vi "Scripts.vi"() -> ()   [LabVIEW 2013]
uses:
  <vilib>/Platform/TimedLoop/XDataNode/wakeup.ctl
  <vilib>/Platform/TimedLoop/XDataNode/XDNodeRunTimeDep.lvlib
  <vilib>/Platform/TimedLoop/XDataNode/nitl_modes.ctl
  <vilib>/Platform/TimedLoop/XDataNode/timing_clust.ctl
  <vilib>/Platform/TimedLoop/XDataNode/XDataNode.xnode
panel:
  in  "Stop All":bool=TRUE
  in  "Green Laser ON/Interlacing":bool
  in  "Green laser mode":enum32{"Laser ON", "Laser OFF", "Interlace"}(radio)
  in  "Green FB On/Off":bool
  in  "Stop Saving":bool
  in  "Fl. Triggered...":bool
  out "Tether":bool
  in  "Save ave N":dbl=500.0 caption="Averaging Factor"
  out "Raster Scanning...":bool
  out "Saving...":bool
  out "Stage Moving":bool
  in  "Take Detection Laser\nImage":bool
  in  "Step Size (nm)":dbl=0.34
  in  "N Steps":dbl=20.0
  in  "Take Stepping Data":bool
  in  "Save ave factor":dbl=1.0
  in  "Got DNA bead":bool
  in  "Got ADig bead":bool
  in  "Y change (mm)":dbl
  in  "Dip for Protein":bool
  in  "Save Data After?":bool
  in  "Green ON After?":bool
  in  "Dip Trap Delta 2 (MHz)":dbl=15.0
  in  "Move Trap After?":bool
  in  "Duration (s)":dbl=1.0
  in  "Move Trap Before?":bool
  in  "Dip Trap Delta 1 (MHz)":dbl=15.0
  in  "Dump Beads":bool
  in  "Cal/Data Acq. Spot":bool
  in  "Offset 2 Start (MHz)":dbl=16.0
  in  "Offset 2 Set":dbl=2.0
  in  "Cal read wait (s)":u32=5
  in  "W/ Offset 2":bool
  in  "Offset 1 Start (MHz)":dbl=13.0
  in  "Offset 1 Set":dbl=1.0
  in  "W/ Offset 1":bool=TRUE
  in  "Cal @ (MHz)":dbl=20.0
  in  "Cap 1 T ON":bool=TRUE
  in  "Cap 1 Flow ON":bool=TRUE
  in  "Move Cap. 1 (DNA Top)":bool
  in  "Cap 1 Samp Flow ON":bool=TRUE
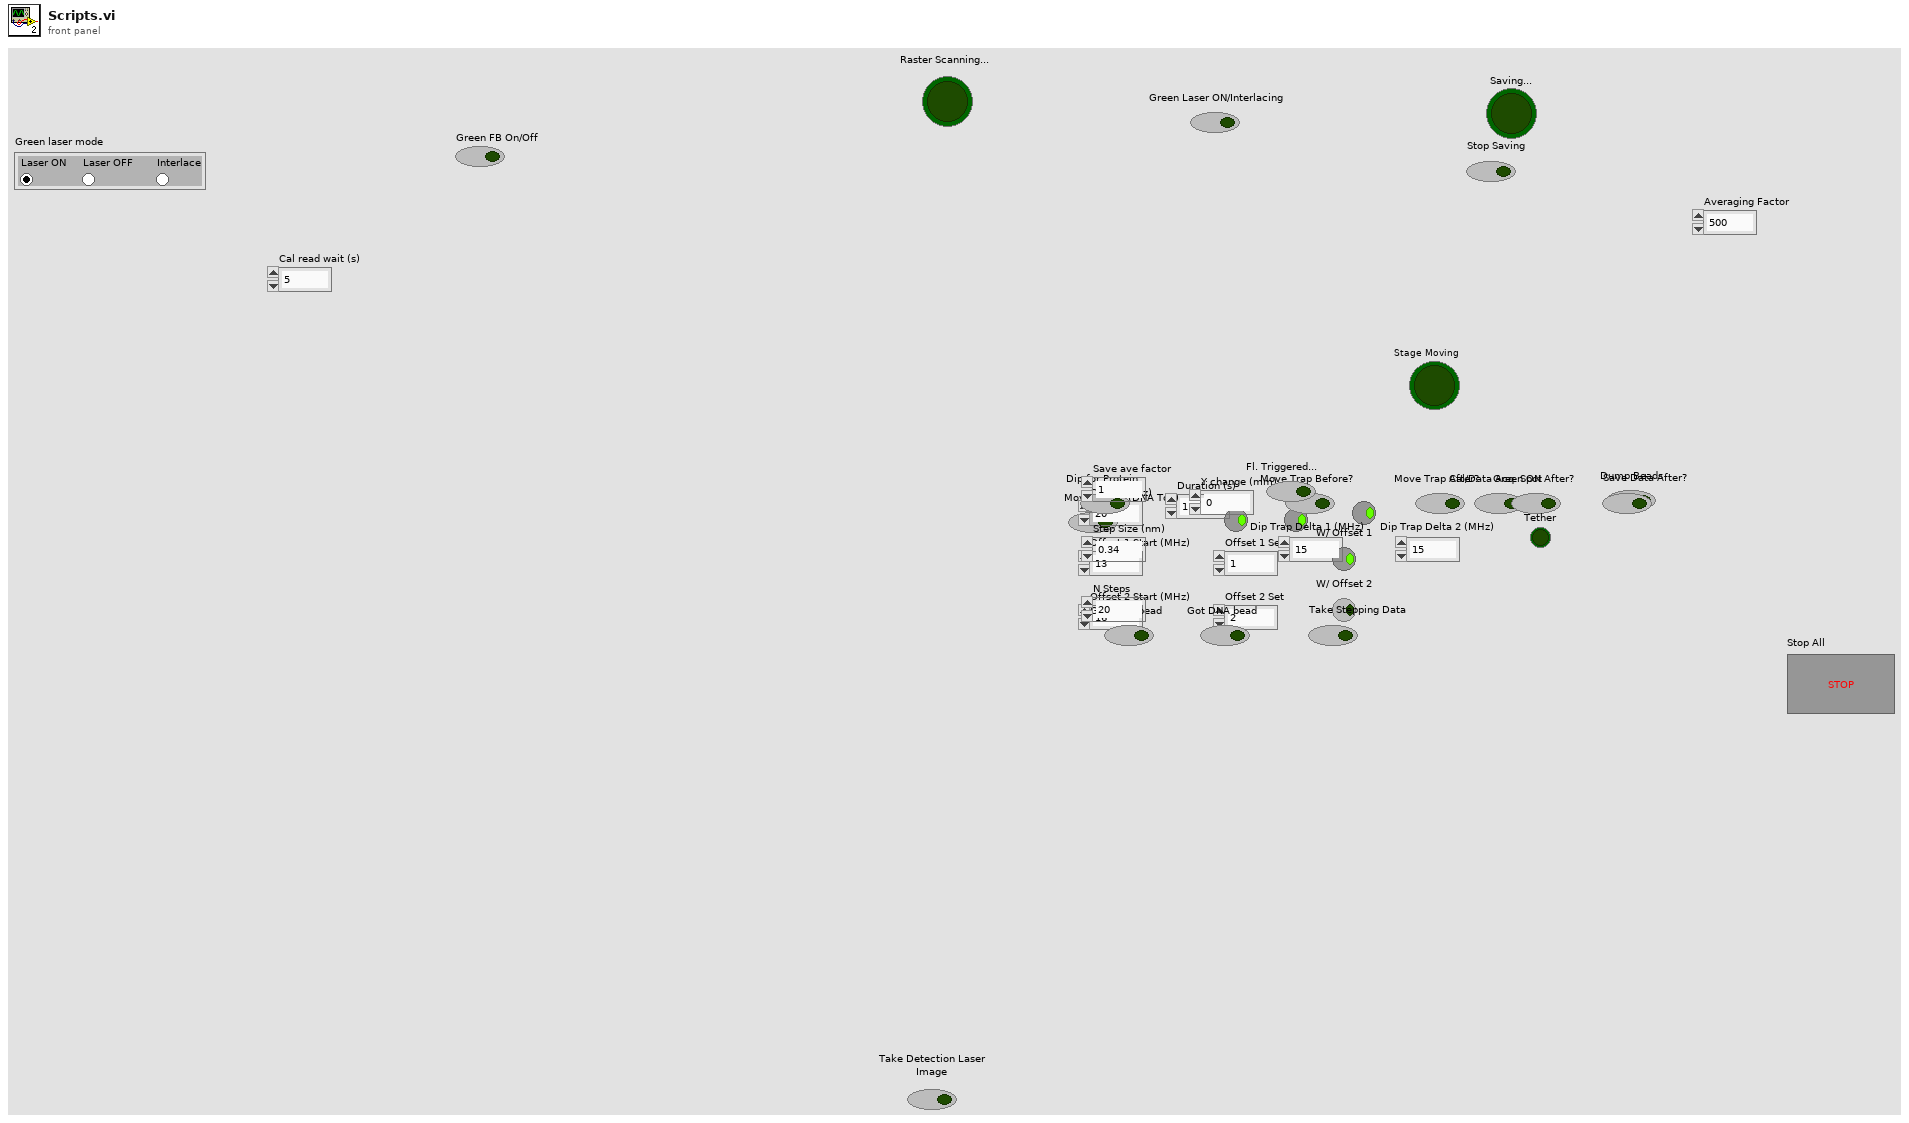
[diagram p1: front panel]
types:
  T1 = typedef "XDNodeRunTimeDep.lvlib/timing_clust.ctl" = cluster{"Expected End [f-1]":u64, "Actual End [f-1]":u64, "Finished Late? [f-1]":bool, "Expected End [i-1]":u64, "Actual End [i-1]":u64, "Finished Late? [i-1]":bool, "Expected Start [i]":u64, "Actual Start [i]":u64, "Expected Start [f]":u64, "Actual Start [f]":u64, "Source Name":string, "Structure Name":string, "Period":i64, "Deadline":i64, "Offset":i64, "Start":i64, "Priority":i32, "Timeout":i32, "Mode":T2, "Wakeup Reason":T3, "Error":errorcluster, "Source Type":string, "Secondary Source Type":string, "Global End Time":u64, "Global Start Time":u64, "Frame Duration":u64, "Iteration Duration":u64, "Assigned CPU":i32, "I/O Scan Engine Mode":u32}
  T2 = typedef "XDNodeRunTimeDep.lvlib/nitl_modes.ctl" = enum32{"No Change", "Process missed periods, maintain original phase", "Discard missed periods, maintain original phase", "Process missed periods, ignore original phase", "Discard missed periods, ignore original phase"}
  T3 = typedef "XDNodeRunTimeDep.lvlib/wakeup.ctl" = enum32{"Normal", "Aborted", "Asynchronous wakeup", "Timing source error", "Timed loop error", "Timeout"}
  T4 = enum16{"CONNECT", "INITIALIZE VALVES", "DISCONNECT", "MOVE VALVE"}
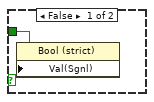
[diagram p4: hidden frame]
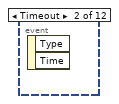
[diagram p5: hidden frame]
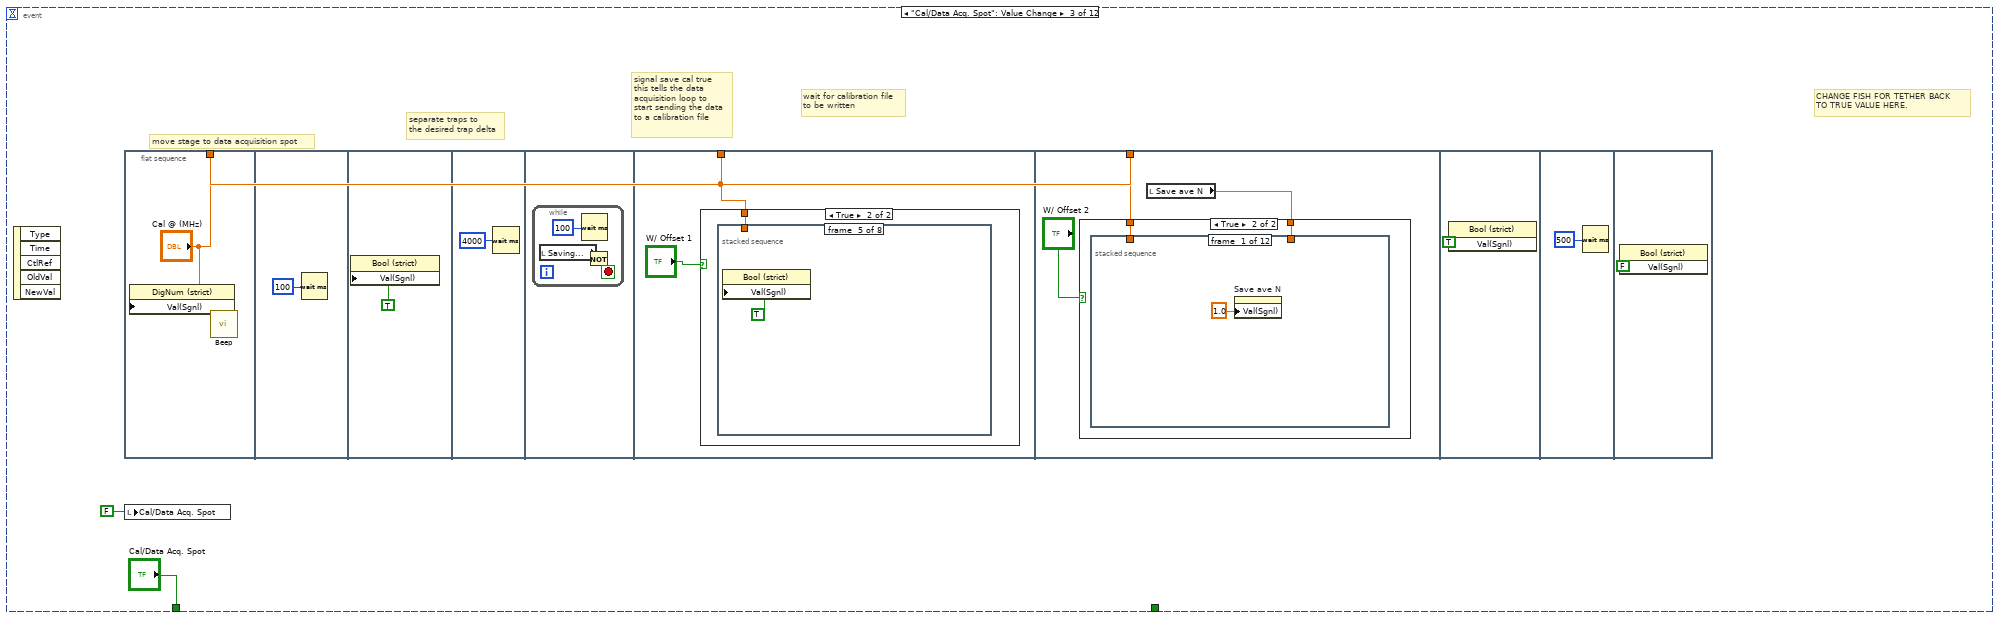
[diagram p6: hidden frame]
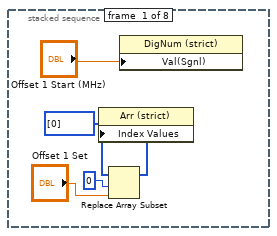
[diagram p8: hidden frame]
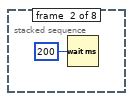
[diagram p9: hidden frame]
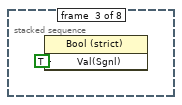
[diagram p10: hidden frame]
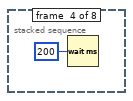
[diagram p11: hidden frame]
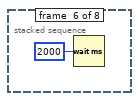
[diagram p12: hidden frame]
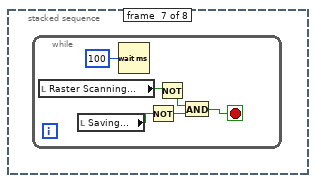
[diagram p13: hidden frame]
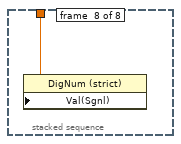
[diagram p14: hidden frame]
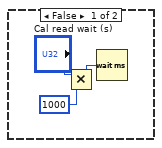
[diagram p15: hidden frame]
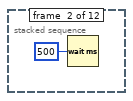
[diagram p16: hidden frame]
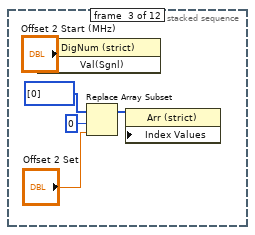
[diagram p17: hidden frame]
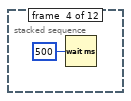
[diagram p18: hidden frame]
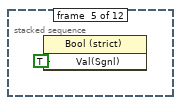
[diagram p19: hidden frame]
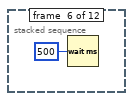
[diagram p20: hidden frame]
diagram:
  n1 = node-c288() -> (w2:T1)  [unwired: 4 in]
  n2 = timed-loop "Run Scripts, including: stage motion" {
    timing: w2 -> [_]
    timing-out: [_] -> w1
    stop <- w4 stop-if-true
    n3 = node-c288() -> ()  [unwired: 1 in, 1 out]
    n4 = event shown="[0] \"Move Cap. 1 (DNA Top)\": Value Change" {
      selector: _ -> [_ _ _ _ _ _ _ _ _ _ _ _]
      dyn-events: _ -> [_ _ _ _ _ _ _ _ _ _ _ _]
      timeout: 50 -> [_ _ _ _ _ _ _ _ _ _ _ _]
      tunnel: ["Move Cap. 1 (DNA Top)" _ "Cal/Data Acq. Spot" "Dump Beads" "Dip for Protein" _ "Got ADig bead" "Got DNA bead" "Take Stepping Data" _ "Take Detection Laser\nImage" _] -> _
      tunnel: [_ _ _ _ _ _ _ _ _ _ _ w212] -> w4
      event "Move Cap. 1 (DNA Top)": Value Change {
        n5 = event-data() -> ()  [unwired: 1 in, 5 out]
        n6 = local write "Move Cap. 1 (DNA Top)"(FALSE ("Move Cap. 1 (DNA Right)")) -> ()
        n7 = flat-sequence {
          tunnel: "Cap 1 Samp Flow ON" -> [w10]
          frame #0 {
            n8 = local write "Stage Moving"(FALSE ("Stage Moving")) -> ()
            n9 = case "stop flow" shown="True" w10 {
              frame False {
              }
              frame True {
                n10 = call "hamilton_controller.vi"("Open?"=FALSE, "valve"=enum16{"A", "B", "C", "D", "ALL"}."C", "action"=T4."MOVE VALVE") -> ()  [unwired: 8 in, 1 out]
              }
            }
            n11 = case shown="True" TRUE {
              tunnel: "Cap 1 T ON" -> [w19 w20]
              frame False {
                n12 = property on="Property Node" class="Bool (strict)"("Val(Sgnl)"=w19) -> ()  [unwired: 2 in, 2 out]
              }
              frame True {
                n13 = property on="Property Node" class="Bool (strict)"("Val(Sgnl)"=w20) -> ()  [unwired: 2 in, 2 out]
              }
            }
            n14 = call <vilib>:"Beep.vi"() -> ()  [unwired: 3 in, 9 out]
            n15 = case shown="True" "Cap 1 Flow ON" {
              frame False {
              }
              frame True {
                n16 = property on="Property Node" class="Bool (strict)"("Val(Sgnl)"=TRUE ("Value (Signaling)")) -> ()  [unwired: 2 in, 2 out]
              }
            }
          }
        }
      }
      event Timeout {
        n17 = event-data() -> ()  [unwired: 1 in, 2 out]
      }
      event "Cal/Data Acq. Spot": Value Change {
        # "wait for calibration file\nto be written"
        # "signal save cal true\nthis tells the data \nacquisition loop to\nstart sending the data\nto a calibration file"
        # "separate traps to\nthe desired trap delta"
        # "move stage to data acquisition spot"
        # "CHANGE FISH FOR TETHER BACK\nTO TRUE VALUE HERE."
        n18 = event-data() -> ()  [unwired: 1 in, 5 out]
        n19 = flat-sequence {
          tunnel: ["Cal @ (MHz)"] -> w21
          tunnel: w21 -> [w31]
          tunnel: w21 -> [w52]
          frame #0 {
            n20 = property on="Property Node" class="DigNum (strict)"("Val(Sgnl)"="Cal @ (MHz)") -> ()  [unwired: 2 in, 2 out]
            n21 = call <vilib>:"Beep.vi"() -> ()  [unwired: 3 in, 9 out]
          }
          frame #1 {
            n22 = Wait (ms)(milliseconds to wait=u32 100) -> ()  [unwired: 1 out]
          }
          frame #2 {
            n23 = property on="Property Node" class="Bool (strict)"("Val(Sgnl)"=TRUE ("Value (Signaling)")) -> ()  [unwired: 2 in, 2 out]
          }
          frame #3 {
            n24 = Wait (ms)(milliseconds to wait=u32 4000) -> ()  [unwired: 1 out]
          }
          frame #4 {
            n25 = while {
              stop <- w28 stop-if-true
              n26 = local read "Saving..."() -> (w29:bool)
              n27 = Wait (ms)(milliseconds to wait=u32 100) -> ()  [unwired: 1 out]
              n28 = Not(x=w29) -> (.not. x?=w28:bool)
            }
          }
          frame #5 {
            n29 = case shown="True" "W/ Offset 1" {
              tunnel: w31 -> [_ w33]
              frame False {
              }
              frame True {
                n30 = stacked-sequence {
                  tunnel: w33 -> [_ _ _ _ _ _ _ w50]
                  frame #0 {
                    n31 = Replace Array Subset(array=u32[] [0] ("Index Values"), new element="Offset 1 Set", index=0) -> (w34:u32[])
                    n32 = property on="Property Node" class="Arr (strict)"("Index Values"=w34) -> ()  [unwired: 2 in, 2 out]
                    n33 = property on="Property Node" class="DigNum (strict)"("Val(Sgnl)"="Offset 1 Start (MHz)") -> ()  [unwired: 2 in, 2 out]
                  }
                  frame #1 {
                    n34 = Wait (ms)(milliseconds to wait=u32 200) -> ()  [unwired: 1 out]
                  }
                  frame #2 {
                    n35 = property on="Property Node" class="Bool (strict)"("Val(Sgnl)"=TRUE ("Value (Signaling)")) -> ()  [unwired: 2 in, 2 out]
                  }
                  frame #3 {
                    n36 = Wait (ms)(milliseconds to wait=u32 200) -> ()  [unwired: 1 out]
                  }
                  frame #4 {
                    n37 = property on="Property Node" class="Bool (strict)"("Val(Sgnl)"=TRUE ("Value (Signaling)")) -> ()  [unwired: 2 in, 2 out]
                  }
                  frame #5 {
                    n38 = Wait (ms)(milliseconds to wait=u32 2000) -> ()  [unwired: 1 out]
                  }
                  frame #6 {
                    n39 = while {
                      stop <- w47 stop-if-true
                      n40 = local read "Raster Scanning..."() -> (w49:bool)
                      n41 = local read "Saving..."() -> (w45:bool)
                      n42 = Wait (ms)(milliseconds to wait=u32 100) -> ()  [unwired: 1 out]
                      n43 = Not(x=w45) -> (.not. x?=w44:bool)
                      n44 = Not(x=w49) -> (.not. x?=w46:bool)
                      n45 = And(x=w46, y=w44) -> (x .and. y?=w47:bool)
                    }
                  }
                  frame #7 {
                    n46 = property on="Property Node" class="DigNum (strict)"("Val(Sgnl)"=w50) -> ()  [unwired: 2 in, 2 out]
                  }
                }
              }
            }
          }
          frame #6 {
            n47 = local read "Save ave N"() -> (w51:dbl)
            n48 = case shown="True" "W/ Offset 2" {
              tunnel: w52 -> [_ w58]
              tunnel: w51 -> [_ w57]
              frame False {
                n49 = Multiply(x="Cal read wait (s)", y=u32 1000 ("milliseconds to wait")) -> (x*y=w55:u32)
                n50 = Wait (ms)(milliseconds to wait=w55) -> ()  [unwired: 1 out]
              }
              frame True {
                n51 = stacked-sequence {
                  tunnel: w58 -> [_ _ _ _ _ _ _ _ _ w79 _ _]
                  tunnel: w57 -> [_ _ _ _ _ _ _ _ _ w77 _ _]
                  frame #0 {
                    n52 = property on="Save ave N" class="DigNum (strict)"("Val(Sgnl)"=1.0 ("Value (Signaling)")) -> ()  [unwired: 2 in, 2 out]
                  }
                  frame #1 {
                    n53 = Wait (ms)(milliseconds to wait=u32 500) -> ()  [unwired: 1 out]
                  }
                  frame #2 {
                    n54 = property on="Property Node" class="DigNum (strict)"("Val(Sgnl)"="Offset 2 Start (MHz)") -> ()  [unwired: 2 in, 2 out]
                    n55 = Replace Array Subset(array=u32[] [0] ("Index Values"), new element="Offset 2 Set", index=0) -> (w63:u32[])
                    n56 = property on="Property Node" class="Arr (strict)"("Index Values"=w63) -> ()  [unwired: 2 in, 2 out]
                  }
                  frame #3 {
                    n57 = Wait (ms)(milliseconds to wait=u32 500) -> ()  [unwired: 1 out]
                  }
                  frame #4 {
                    n58 = property on="Property Node" class="Bool (strict)"("Val(Sgnl)"=TRUE ("Value (Signaling)")) -> ()  [unwired: 2 in, 2 out]
                  }
                  frame #5 {
                    n59 = Wait (ms)(milliseconds to wait=u32 500) -> ()  [unwired: 1 out]
                  }
                  frame #6 {
                    n60 = property on="Property Node" class="Bool (strict)"("Val(Sgnl)"=TRUE ("Value (Signaling)")) -> ()  [unwired: 2 in, 2 out]
                  }
                  frame #7 {
                    n61 = Wait (ms)(milliseconds to wait=u32 2000) -> ()  [unwired: 1 out]
                  }
                  frame #8 {
                    n62 = while {
                      stop <- w72 stop-if-true
                      n63 = local read "Raster Scanning..."() -> (w75:bool)
                      n64 = local read "Saving..."() -> (w73:bool)
                      n65 = Wait (ms)(milliseconds to wait=u32 100) -> ()  [unwired: 1 out]
                      n66 = Not(x=w73) -> (.not. x?=w71:bool)
                      n67 = Not(x=w75) -> (.not. x?=w74:bool)
                      n68 = And(x=w74, y=w71) -> (x .and. y?=w72:bool)
                    }
                  }
                  frame #9 {
                    n69 = property on="Property Node" class="DigNum (strict)"("Val(Sgnl)"=w79) -> ()  [unwired: 2 in, 2 out]
                    n70 = property on="Property Node" class="Arr (strict)"("Index Values"=u32[] [0]) -> ()  [unwired: 2 in, 2 out]
                    n71 = property on="Save ave N" class="DigNum (strict)"("Val(Sgnl)"=w77) -> ()  [unwired: 2 in, 2 out]
                  }
                  frame #10 {
                    n72 = Wait (ms)(milliseconds to wait=u32 500) -> ()  [unwired: 1 out]
                  }
                  frame #11 {
                    n73 = property on="Property Node" class="Bool (strict)"("Val(Sgnl)"=TRUE ("Value (Signaling)")) -> ()  [unwired: 2 in, 2 out]
                  }
                }
              }
            }
          }
          frame #7 {
            n74 = property on="Property Node" class="Bool (strict)"("Val(Sgnl)"=TRUE ("Value (Signaling)")) -> ()  [unwired: 2 in, 2 out]
          }
          frame #8 {
            n75 = Wait (ms)(milliseconds to wait=u32 500) -> ()  [unwired: 1 out]
          }
          frame #9 {
            n76 = property on="Property Node" class="Bool (strict)"("Val(Sgnl)"=FALSE ("Value (Signaling)")) -> ()  [unwired: 2 in, 2 out]
          }
        }
        n77 = local write "Cal/Data Acq. Spot"(FALSE ("Cal/Data Acq. Spot")) -> ()
      }
      event "Dump Beads": Value Change {
        # "SCRIPT TO REMOVE BOTH BEADS FROM THE TRAPS. TURNS ON LIGHT WHICH INDICATES THAT STAGE IS MOVING. THEN STOPS SAVING DATA. \nSETS Sample Channel Flow TO TRUE. STOPS INTERLACING GREEN FLUORESCENCE. TURNS OFF Tether INDICATOR BECAUSE WE ARE THROWING IT\nAWAY. SHUTS OFF TRAP POSITION FEEDBACK."
        n78 = event-data() -> ()  [unwired: 1 in, 5 out]
        n79 = flat-sequence {
          frame #0 {
            w86 = FALSE ("Fl. Triggered...")
            w87 = TRUE ("Stage Moving")
            n80 = local read "Saving..."() -> (w88:bool)
            n81 = property on="Property Node" class="Bool (strict)"("Val(Sgnl)"=w86) -> ()  [unwired: 2 in, 2 out]
            n82 = local write "Fl. Triggered..."(w86) -> ()
            n83 = local write "Stage Moving"(w87) -> ()
            n84 = local write "Tether"(w86) -> ()
            n85 = property on="Property Node" class="Bool (strict)"("Val(Sgnl)"=w87) -> ()  [unwired: 2 in, 2 out]
            n86 = property on="Green Laser ON/Interlacing" class="Bool (strict)"("Val(Sgnl)"=w86) -> ()  [unwired: 2 in, 2 out]
            n87 = local write "Stop Saving"(w88) -> ()
          }
          frame #1 {
            w89 = FALSE ("Value (Signaling)")
            # "TURNS TRAPS OFF SO THAT\nBEADS REMAIN AT DUMP \nBEADS POSITION"
            n88 = property on="Property Node" class="Bool (strict)"("Val(Sgnl)"=w89) -> ()  [unwired: 2 in, 2 out]
            n89 = property on="Property Node" class="Bool (strict)"("Val(Sgnl)"=w89) -> ()  [unwired: 2 in, 2 out]
            n90 = call <vilib>:"Beep.vi"() -> ()  [unwired: 3 in, 9 out]
          }
          frame #2 {
            w90 = TRUE ("Value (Signaling)")
          }
          frame #3 {
            n91 = Wait (ms)(milliseconds to wait=u32 8000) -> ()  [unwired: 1 out]
          }
          frame #4 {
            n92 = property on="Property Node" class="DigNum (strict)"("Val(Sgnl)"=20.0 ("Value (Signaling)")) -> ()  [unwired: 2 in, 2 out]
          }
          frame #5 {
            n93 = property on="Property Node" class="Bool (strict)"("Val(Sgnl)"=TRUE ("Value (Signaling)")) -> ()  [unwired: 2 in, 2 out]
          }
          frame #6 {
            n94 = property on="Property Node" class="Bool (strict)"("Val(Sgnl)"=FALSE ("Value (Signaling)")) -> ()  [unwired: 2 in, 2 out]
          }
        }
      }
      event "Dip for Protein": Value Change {
        n95 = event-data() -> ()  [unwired: 1 in, 5 out]
        n96 = flat-sequence {
          frame #0 {
            n97 = case shown="True" "Move Trap Before?" {
              frame False {
              }
              frame True {
                n98 = property on="Property Node" class="DigNum (strict)"("Val(Sgnl)"="Dip Trap Delta 1 (MHz)") -> ()  [unwired: 2 in, 2 out]
              }
            }
          }
          frame #1 {
            n99 = Multiply(x="Duration (s)", y=1000.0) -> (x*y=w98:dbl)
            n100 = Wait (ms)(milliseconds to wait=w98) -> ()  [unwired: 1 out]
          }
          frame #2 {
            n101 = case shown="True" "Move Trap After?" {
              frame False {
              }
              frame True {
                n102 = property on="Property Node" class="DigNum (strict)"("Val(Sgnl)"="Dip Trap Delta 2 (MHz)") -> ()  [unwired: 2 in, 2 out]
              }
            }
          }
          frame #3 {
            n103 = case shown="True" "Green ON After?" {
              frame False {
              }
              frame True {
                n104 = property on="Green Laser ON/Interlacing" class="Bool (strict)"("Val(Sgnl)"=TRUE ("Value (Signaling)")) -> ()  [unwired: 2 in, 2 out]
              }
            }
          }
          frame #4 {
            n105 = Wait (ms)(milliseconds to wait=u32 500) -> ()  [unwired: 1 out]
          }
          frame #5 {
            n106 = case shown="True" "Save Data After?" {
              frame False {
              }
              frame True {
                n107 = property on="Property Node" class="Bool (strict)"("Val(Sgnl)"=TRUE ("Value (Signaling)")) -> ()  [unwired: 2 in, 2 out]
              }
            }
          }
        }
      }
      event #5 (no event record) {
        n108 = event-data() -> ()  [unwired: 1 in, 5 out]
        n109 = flat-sequence {
          frame #0 {
            w108 = 0.0 ("element")
            n110 = Build Array(w108, "Y change (mm)", w108) -> ()  [unwired: 1 out]
          }
          frame #1 {
            # "stop saving"
            n111 = local write "Stop Saving"(TRUE ("Stop Saving")) -> ()
            n112 = local write "Stage Moving"(FALSE ("Stage Moving")) -> ()
          }
        }
      }
      event "Got ADig bead": Value Change {
        n113 = event-data() -> ()  [unwired: 1 in, 5 out]
        n114 = property on="Property Node" class="Bool (strict)"("Val(Sgnl)"=FALSE ("Value (Signaling)")) -> ()  [unwired: 2 in, 2 out]
        n115 = property on="Move Cap. 1 (DNA Top)" class="Bool (strict)"("Val(Sgnl)"=TRUE ("Value (Signaling)")) -> ()  [unwired: 2 in, 2 out]
      }
      event "Got DNA bead": Value Change {
        n116 = event-data() -> ()  [unwired: 1 in, 5 out]
        n117 = property on="Property Node" class="Bool (strict)"("Val(Sgnl)"=FALSE ("Value (Signaling)")) -> ()  [unwired: 2 in, 2 out]
        n118 = property on="Cal/Data Acq. Spot" class="Bool (strict)"("Val(Sgnl)"=TRUE ("Value (Signaling)")) -> ()  [unwired: 2 in, 2 out]
      }
      event "Take Stepping Data": Value Change {
        n119 = event-data() -> ()  [unwired: 1 in, 5 out]
        n120 = local read "Save ave N"() -> (w126:dbl)
        n121 = flat-sequence {
          tunnel: w126 -> [w128]
          tunnel: [w128] -> w121
          tunnel: [w130] -> w122
          tunnel: w121 -> [w130]
          tunnel: [w132] -> w123
          tunnel: w122 -> [w132]
          tunnel: [w135] -> w124
          tunnel: w123 -> [w135]
          tunnel: [w137] -> w125
          tunnel: w124 -> [w137]
          tunnel: [w139] -> w119
          tunnel: w125 -> [w139]
          tunnel: w119 -> [w142]
          tunnel: [w142] -> w118
          tunnel: w118 -> [w143]
          tunnel: [w143] -> w120
          tunnel: w120 -> [w149]
          frame #0 {
            n122 = property on="Save ave N" class="DigNum (strict)"("Val(Sgnl)"="Save ave factor") -> ()  [unwired: 2 in, 2 out]
          }
          frame #1 {
            n123 = Wait (ms)(milliseconds to wait=u32 100) -> ()  [unwired: 1 out]
          }
          frame #2 {
            n124 = local read "Offset 2 Start (MHz)"() -> (w134:dbl)
            n125 = property on="Property Node" class="Arr (strict)"("Index Values"=u32[] [2]) -> ()  [unwired: 2 in, 2 out]
            n126 = property on="Property Node" class="DigNum (strict)"("Val(Sgnl)"=w134) -> ()  [unwired: 2 in, 2 out]
          }
          frame #3 {
            n127 = property on="Property Node" class="Bool (strict)"("Val(Sgnl)"=TRUE ("Value (Signaling)")) -> ()  [unwired: 2 in, 2 out]
          }
          frame #4 {
            n128 = Wait (ms)(milliseconds to wait=u32 100) -> ()  [unwired: 1 out]
          }
          frame #5 {
            n129 = property on="Property Node" class="Bool (strict)"("Val(Sgnl)"=TRUE ("Value (Signaling)")) -> ()  [unwired: 2 in, 2 out]
          }
          frame #6 {
            n130 = Wait (ms)(milliseconds to wait=u32 1000) -> ()  [unwired: 1 out]
          }
          frame #7 {
            n131 = while {
              stop <- w146 stop-if-true
              n132 = local read "Raster Scanning..."() -> (w148:bool)
              n133 = local read "Saving..."() -> (w147:bool)
              n134 = Not(x=w147) -> (.not. x?=w144:bool)
              n135 = Not(x=w148) -> (.not. x?=w145:bool)
              n136 = And(x=w145, y=w144) -> (x .and. y?=w146:bool)
            }
          }
          frame #8 {
            n137 = property on="Save ave N" class="DigNum (strict)"("Val(Sgnl)"=w149) -> ()  [unwired: 2 in, 2 out]
          }
        }
      }
      event "Step Size (nm)": Value Change {
        n138 = event-data() -> ()  [unwired: 1 in, 5 out]
        n139 = flat-sequence {
          frame #0 {
            n140 = property on="Property Node" class="Arr (strict)"("Index Values"=u32[] [1]) -> ()  [unwired: 2 in, 2 out]
          }
          frame #1 {
            n141 = property on="Property Node" class="DigNum (strict)"("Value"="Step Size (nm)") -> ()  [unwired: 2 in, 2 out]
            n142 = property on="Property Node" class="DigNum (strict)"("Value"="Step Size (nm)") -> ()  [unwired: 2 in, 2 out]
            n143 = Multiply(x="N Steps", y="Step Size (nm)") -> (x*y=w151:dbl)
            n144 = property on="Property Node" class="DigNum (strict)"("Value"=w151) -> ()  [unwired: 2 in, 2 out]
          }
        }
      }
      event "Take Detection Laser\nImage": Value Change {
        n145 = event-data() -> ()  [unwired: 1 in, 5 out]
        n146 = flat-sequence {
          tunnel: [w179] -> w169
          tunnel: [w178] -> w162
          tunnel: [w177] -> w154
          tunnel: [w182] -> w170
          tunnel: w169 -> [w182]
          tunnel: [w181] -> w163
          tunnel: w162 -> [w181]
          tunnel: [w180] -> w155
          tunnel: w154 -> [w180]
          tunnel: [w186] -> w171
          tunnel: w170 -> [w186]
          tunnel: [w185] -> w164
          tunnel: w163 -> [w185]
          tunnel: [w184] -> w156
          tunnel: w155 -> [w184]
          tunnel: [w192] -> w172
          tunnel: w171 -> [w192]
          tunnel: [w191] -> w165
          tunnel: w164 -> [w191]
          tunnel: [w190] -> w157
          tunnel: w156 -> [w190]
          tunnel: [w196] -> w173
          tunnel: w172 -> [w196]
          tunnel: [w195] -> w166
          tunnel: w165 -> [w195]
          tunnel: [w194] -> w158
          tunnel: w157 -> [w194]
          tunnel: [w200] -> w174
          tunnel: w173 -> [w200]
          tunnel: [w199] -> w167
          tunnel: w166 -> [w199]
          tunnel: [w198] -> w159
          tunnel: w158 -> [w198]
          tunnel: [w204] -> w175
          tunnel: w174 -> [w204]
          tunnel: [w203] -> w168
          tunnel: w167 -> [w203]
          tunnel: [w202] -> w160
          tunnel: w159 -> [w202]
          tunnel: w175 -> [w210]
          tunnel: w168 -> [w209]
          tunnel: [w207] -> w161
          tunnel: w160 -> [w207]
          tunnel: w161 -> [w211]
          frame #0 {
            n147 = local read "Green Laser ON/Interlacing"() -> (w179:bool)
            n148 = local read "Green laser mode"() -> (w178:enum32{"Laser ON", "Laser OFF", "Interlace"})
            n149 = local read "Green FB On/Off"() -> (w177:bool)
          }
          frame #1 {
            n150 = property on="Green FB On/Off" class="Bool (strict)"("Val(Sgnl)"=FALSE ("Value (Signaling)")) -> ()  [unwired: 2 in, 2 out]
          }
          frame #2 {
            n151 = property on="Property Node" class="Bool (strict)"("Val(Sgnl)"=TRUE ("Value (Signaling)")) -> ()  [unwired: 2 in, 2 out]
            n152 = property on="Green Laser ON/Interlacing" class="Bool (strict)"("Val(Sgnl)"=TRUE ("Value (Signaling)")) -> ()  [unwired: 2 in, 2 out]
            n153 = property on="Green laser mode" class="RadioBtnsControl (strict)"("Val(Sgnl)"=enum32{"Laser ON", "Laser OFF", "Interlace"}."Laser ON" ("Value (Signaling)")) -> ()  [unwired: 2 in, 2 out]
          }
          frame #3 {
            n154 = Wait (ms)(milliseconds to wait=u32 500) -> ()  [unwired: 1 out]
          }
          frame #4 {
            n155 = property on="Property Node" class="Bool (strict)"("Val(Sgnl)"=TRUE ("Value (Signaling)")) -> ()  [unwired: 2 in, 2 out]
          }
          frame #5 {
            n156 = Wait (ms)(milliseconds to wait=u32 2000) -> ()  [unwired: 1 out]
          }
          frame #6 {
            n157 = while {
              stop <- w205 stop-if-true
              n158 = local read "Saving..."() -> (w206:bool)
              n159 = Not(x=w206) -> (.not. x?=w205:bool)
            }
          }
          frame #7 {
            n160 = property on="Property Node" class="Bool (strict)"("Val(Sgnl)"=TRUE ("Value (Signaling)")) -> ()  [unwired: 2 in, 2 out]
            n161 = property on="Green Laser ON/Interlacing" class="Bool (strict)"("Val(Sgnl)"=w210) -> ()  [unwired: 2 in, 2 out]
            n162 = property on="Green laser mode" class="RadioBtnsControl (strict)"("Val(Sgnl)"=w209) -> ()  [unwired: 2 in, 2 out]
          }
          frame #8 {
            n163 = property on="Green FB On/Off" class="Bool (strict)"("Val(Sgnl)"=w211) -> ()  [unwired: 2 in, 2 out]
          }
        }
      }
      event "Stop All": Value Change {
        n164 = event-data() -> ()  [unwired: 1 in, 5 out]
        n165 = local read "Stop All"() -> (w212:bool)
      }
    }
    n166 = node-c288() -> ()  [unwired: 1 in, 1 out]
  }
  n167 = node-c288(w1) -> ()  [unwired: 1 out]
